vi "GEvt-Generate Remaining States Log.vi"(0 "CSM Global Log Event":T4, 2 "Remaining States":string="<Remaining States>", 6 "Name (\"\" to Use UUID)":string, 7 "Enable?":bool, 10 "CSM:LogFilter.lvclass":refnum<class "LogFilter.lvclass">) -> (14 "CSM Global Log Event Out":T4, 16 "Event Data":T1={"Name (\"\" to Use UUID)"="", "Current State"="", "Arguments"="", "Source Message"={"‘State"="", "’Arguments"="", "’Error"={"status"=FALSE, "code"=0, "source"=""}}, "Source Module"="", "Complete(T)/Start(F)"=FALSE, "LogType"=enum."State Change", "Time Stamp"=timestamp(0 s since 1904-01-01)})   [LabVIEW 2017, in "Communicable State Machine.lvlib"]
doc: "### GEvt-Generate Remaining States Log.vi\n\n-- <b>Controls</b> --\n- <b>CSM Global Log Event</b>:\n- <b>Remaining States</b>:\n- <b>Name(\"\" to use uuid)</b>:\n- <b>Enable?</b>:\n- <b>CSM:LogFilter.lvclass</b>:\n\n-- <b>Indicators</b> --\n- <b>CSM Global Log Event out</b>:\n- <b>event data</b>:"
uses:
  Communicable State Machine.lvlib
  GEvt-Refs.ctl
  Typedef/_CSM_GlobalLog_MSG.ctl
  Typedef/_CSM_Response Source Message.ctl
  Typedef/_CSM_GlobalLog_MSG_TYPE.ctl
  LogFilter/LogFilter.lvclass
  LogFilter/LogFilter - Check.vi
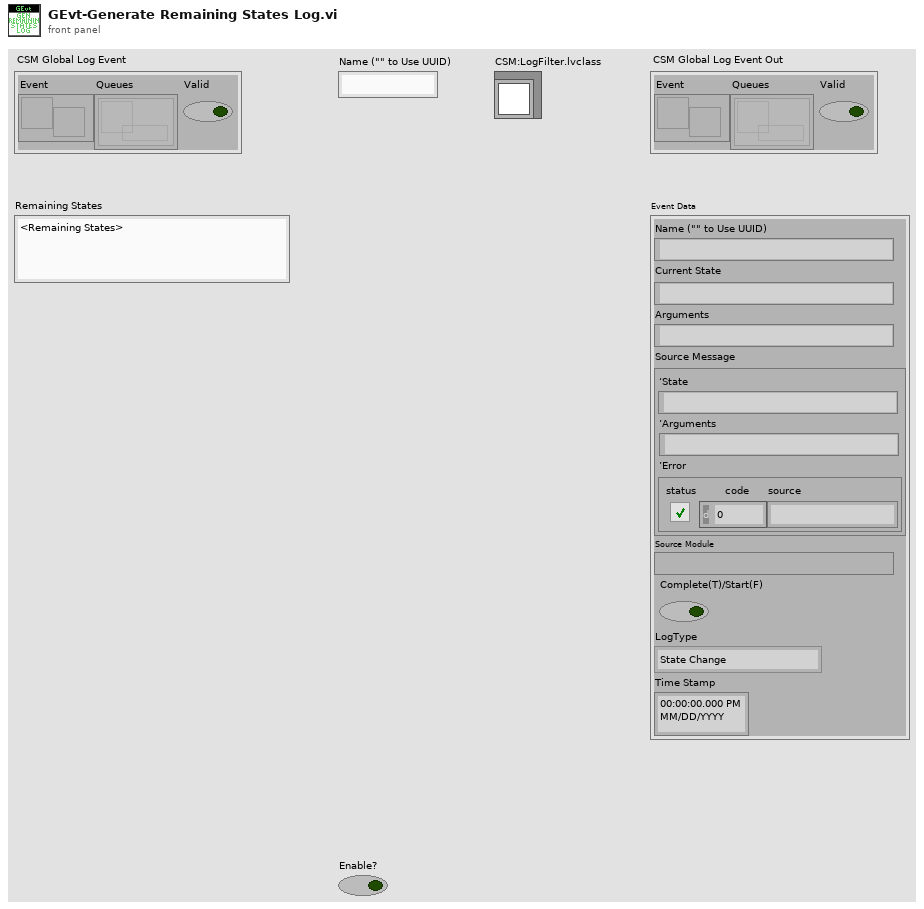
[diagram p1: front panel]
types:
  T1 = typedef "Communicable State Machine.lvlib/_CSM_GlobalLog_MSG.ctl" = cluster{"Name (\"\" to Use UUID)":string, "Current State":string, "Arguments":string, "Source Message":T2, "Source Module":string, "Complete(T)/Start(F)":bool, "LogType":T3, "Time Stamp":timestamp}
  T2 = typedef "Communicable State Machine.lvlib/_CSM_Response Source Message.ctl" = cluster{"‘State":string, "’Arguments":string, "’Error":errorcluster}
  T3 = typedef "Communicable State Machine.lvlib/_CSM_GlobalLog_MSG_TYPE.ctl" = enum16{"User Log", "State Change", "Status", "Interrupt", "Register", "Unregister", "Error Log", "Module Created", "Module Destroyed", "Async Message", "No-Rep Async Message", "Sync Message", "AsyncMsg Complete", "SyncMsg Complete"}
  T4 = typedef "Communicable State Machine.lvlib/GEvt-Refs.ctl" = cluster{"Event":refnum<user-event>, "Queues":refnum<queue>[], "Valid":bool}
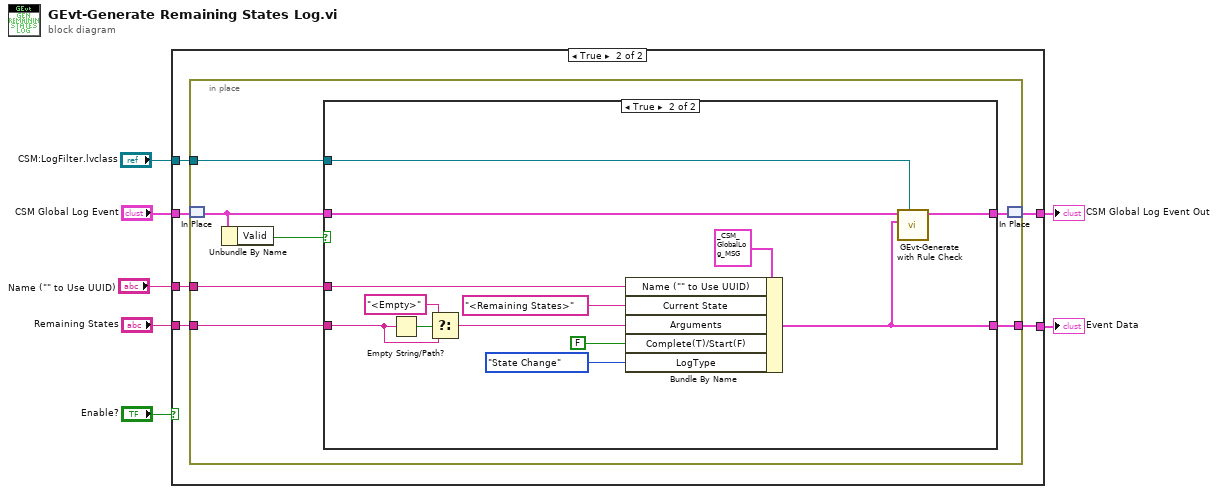
[diagram p0: block diagram]
diagram:
  n1 = case shown="True" "Enable?" {
    tunnel: "CSM Global Log Event" -> [w8 w14]
    tunnel: [w8 w13] -> w6
    tunnel: [_ w12] -> w4
    tunnel: "Name (\"\" to Use UUID)" -> [_ w11]
    tunnel: "Remaining States" -> [_ w10]
    tunnel: "CSM:LogFilter.lvclass" -> [_ w9]
    frame False {
    }
    frame True {
      n2 = in-place {
        in-place-border: [w20] -> w12
        in-place-border: w11 -> [w19]
        in-place-border: w10 -> [w18]
        in-place-border: w9 -> [w17]
        n3 = in-place-match #1(w14) -> (w16:T4)
        n4 = Unbundle By Name(w16) -> ("Valid"=w15:bool)
        n5 = case shown="True" w15 {
          tunnel: w16 -> [w22 w35]
          tunnel: [w22 w34] -> w21
          tunnel: [_ w23] -> w20
          tunnel: w19 -> [_ w26]
          tunnel: w18 -> [_ w25]
          tunnel: w17 -> [_ w24]
          frame False {
          }
          frame True {
            n6 = Empty String/Path?(string/path=w25) -> (empty?=w28:bool)
            n7 = Select(t="<Empty>" ("Current State"), s=w28, f=w25) -> (s? t:f=w27:string)
            n8 = Bundle By Name(cluster=T1 {"Name (\"\" to Use UUID)"="", "Current State"="", "Arguments"="", "Source Message"={"‘State"="", "’Arguments"="", "’Error"={"status"=FALSE, "code"=0, "source"=""}}, "Source Module"="", "Complete(T)/Start(F)"=FALSE, "LogType"=enum."State Change", "Time Stamp"=timestamp(0 s since 1904-01-01)} ("event data"), "Name (\"\" to Use UUID)"=w26, "Current State"="<Remaining States>", "Arguments"=w27, "Complete(T)/Start(F)"=FALSE, "LogType"=_CSM_GlobalLog_MSG_TYPE."State Change" ("Type")) -> (w23:T1)
            n9 = call "GEvt-Generate with Rule Check.vi"("LogFilter In"=w24, "Event Data"=w23, "CSM Global Log Event In"=w35) -> ("CSM Global Log Event Out"=w34:T4)  [unwired: 8 in]
          }
        }
        n10 = in-place-match #1(w21) -> (w13:T4)
      }
    }
  }
  "CSM Global Log Event Out" <- w6
  "Event Data" <- w4
